vi "displayvisexamples.vi"() -> ()   [LabVIEW 2015]
panel:
  in  "stop":bool
  out "error out":errorcluster
  in  "error in (no error)":errorcluster
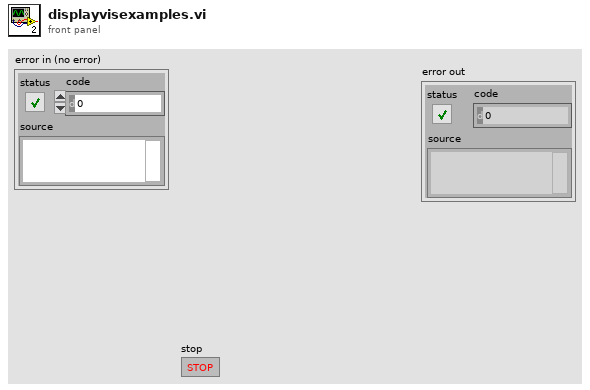
[diagram p1: front panel]
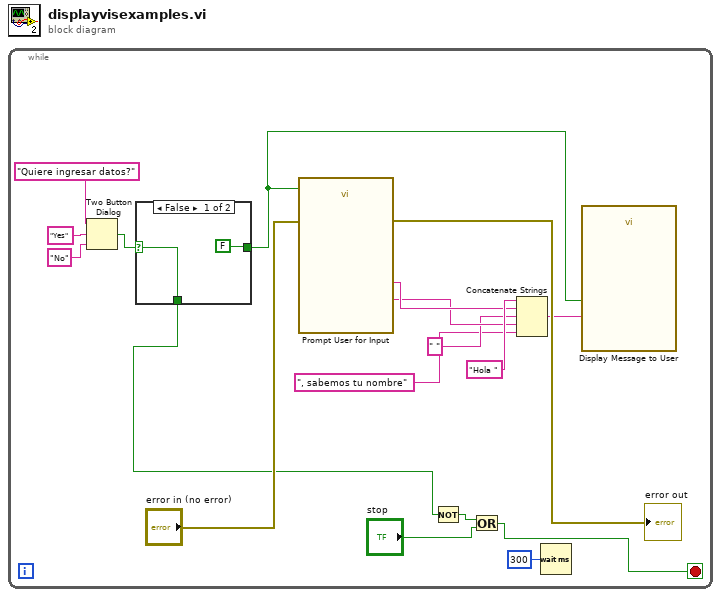
[diagram p0: block diagram]
diagram:
  n1 = while {
    stop <- w4 stop-if-true
    n2 = Two Button Dialog(message="Quiere ingresar datos?", 1:"No" ("F button name (\"Cancel\")"), 2:"Yes" ("T button name (\"OK\")")) -> (T button?=w3:bool)
    n3 = case shown="False" w3 {
      selector: w3 -> [w19 w21]
      tunnel: [FALSE w21] -> w1
      tunnel: [w19 w21] -> w2
      frame False {
      }
      frame True {
      }
    }
    n4 = call "Prompt User for Input"("Enable"=w1, "error in (no error)"="error in (no error)") -> ("Telefono"=w11:string, "Nombre"=w12:string, "error out"=→"error out":errorcluster)  [unwired: 13 in, 2 out]
    n5 = Not(x=w2) -> (.not. x?=w6:bool)
    n6 = Or(x=w6, y="stop") -> (x .or. y?=w4:bool)
    n7 = Concatenate Strings("Hola " ("string"), w12, " " ("string"), w11, ", sabemos tu nombre" ("string")) -> (w8:string)
    n8 = Wait (ms)(milliseconds to wait=u32 300) -> ()  [unwired: 1 out]
    n9 = call "Display Message to User"("Enable"=w1, "Message"=w8) -> ()  [unwired: 8 in, 2 out]
  }
